vi "Switch_Channels2ArrayList.vi"(8 "error in (no error)":errorcluster, 11 "Channel List":string) -> (0 "error out":errorcluster, 3 "Array of Channels":string[](array[string]))   [LabVIEW 2014]
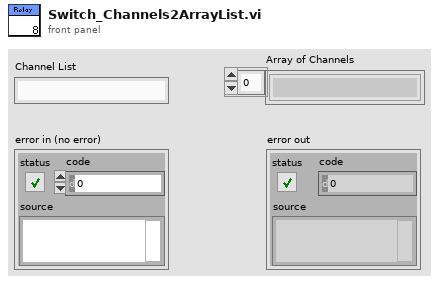
[diagram p1: front panel]
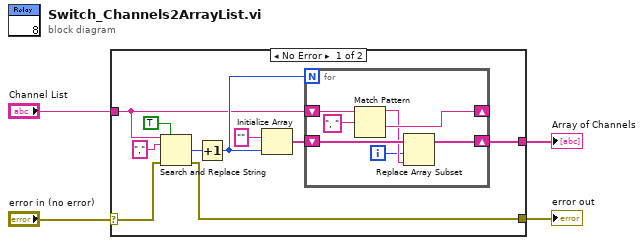
[diagram p0: block diagram]
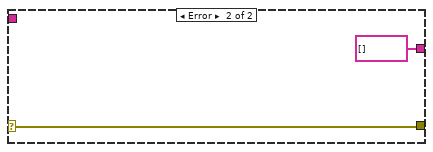
[diagram p2: hidden frame]
diagram:
  n1 = case shown="No Error" "error in (no error)" {
    selector: "error in (no error)" -> [w6 w23]
    tunnel: "Channel List" -> [w8 _]
    tunnel: [w7 string[] []] -> w3
    tunnel: [w5 w23] -> w1
    frame No Error {
      n2 = Search and Replace String(replace all?=TRUE ("replace all? (F)"), input string=w8, search string=",", error in=w6) -> (number of replacements=w11:i32, error out=w5:errorcluster)  [unwired: 4 in, 2 out]
      n3 = Increment(x=w11) -> (x+1=w10:i32)
      n4 = Initialize Array("", w10) -> (w13:string[])
      n5 = for {
        N: w10 -> [_]
        shift-right: [w19] -> _
        shift-left: w8 -> [w21]
        shift-right: [w15] -> w7
        shift-left: w13 -> [w18]
        i -> [w16]
        n6 = Match Pattern(string=w21, regular expression=", ") -> (before substring=w17:string, after substring=w19:string)  [unwired: 1 in, 2 out]
        n7 = Replace Array Subset(array=w18, new element=w17, index=w16) -> (w15:string[])
      }
    }
    frame Error {
    }
  }
  "Array of Channels" <- w3
  "error out" <- w1
